vi "GetRealWorldUnits.vi"(8 "error in (no error)":errorcluster, 11 "XYStage":refnum<class "XYStage.lvclass">) -> (0 "error out":errorcluster, 2 "Real-World Units":string, 3 "XYStage out":refnum<class "XYStage.lvclass">)   [LabVIEW 2015, in "XYStage.lvclass"]
doc: "---------------------------------------------------------------\nJKI State Machine Objects™\nhttp://jki.net/state-machine-objects/\nCopyright (C) 2005-2015, JKI <info@jki.net>\nALL RIGHTS RESERVEDJKI State Machine Objects (SMO) 1.0.0.4\nJKI - JKI\nCopyright (c) 2015, JKI"
uses:
  XYStage.lvclass
panel:
  # "For instructions on how to use the JKI State Machine Objects, examples and video tutorials, visit:\nhttp://jki.net/state-machine-objects/\n\nJKI State Machine Objects™\nhttp://jki.net/state-machine-objects/\nCopyright (C) 2005-2015, JKI <info@jki.net>\nALL RIGHTS RESERVED"
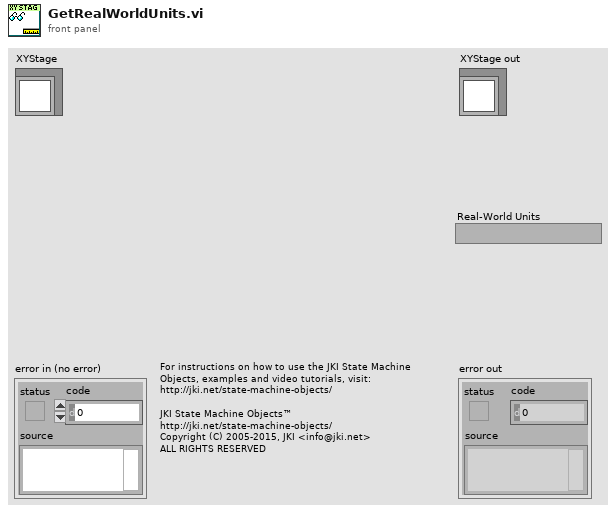
[diagram p1: front panel]
types:
  T1 = typedef "XYStage.lvclass/Configuration--Cluster.ctl" = cluster{"Real-World Units":string, "Counts per Unit":dbl}
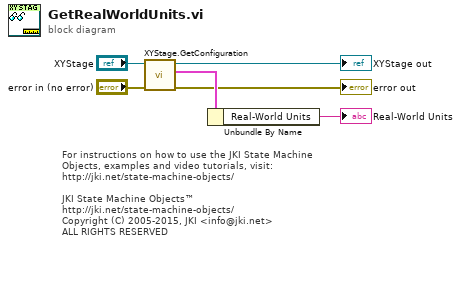
[diagram p0: block diagram]
diagram:
  # "For instructions on how to use the JKI State Machine Objects, examples and video tutorials, visit:\nhttp://jki.net/state-machine-objects/\n\nJKI State Machine Objects™\nhttp://jki.net/state-machine-objects/\nCopyright (C) 2005-2015, JKI <info@jki.net>\nALL RIGHTS RESERVED"
  n1 = call "XYStage.GetConfiguration.vi"("error in (no error)"="error in (no error)", "XYStage"="XYStage") -> ("error out"=→"error out":errorcluster, "Configuration"=w5:T1, "XYStage out"=→"XYStage out":refnum<class "XYStage.lvclass">)  [unwired: 7 in]
  n2 = Unbundle By Name(w5) -> ("Real-World Units"=→"Real-World Units":string)
